vi "Do Core.vi"(8 "error in":errorcluster, 9 "Actor in":refnum<class "Actor.lvclass">, 11 "Reply Message":refnum<class "Get N Images Msg.lvclass">) -> (0 "error out":errorcluster, 1 "Actor out":refnum<class "Actor.lvclass">, 2 "Reply":refnum<class "Generic Image.lvclass">[](array[class]))   [LabVIEW 2024, in "Camera Worker.lvlib" / "Get N Images Msg.lvclass"]
doc: "<p>(<strong>Filename</strong>: <span class=\"dnl\">Actor Framework.lvlib:Reply Msg.lvclass:Do Core.vi</span>)</p>\n<p>Defines what an actor does when it receives <strong>Reply Message</strong>. This method also defines the <strong>Reply</strong> that is returned to the actor that sent <strong>Reply Message</strong>.</p>\n<p>By default, this method does nothing, and <strong>Reply</strong> is the ancestor Message class. A child class must override this method to define behavior and specify a child of the Message class to return in the <strong>Reply</strong> output.</p>"
uses:
  Get N Images Msg.lvclass
  <vilib>/ActorFramework/Actor/Actor.lvclass
  Typedefs/Generic Image/Generic Image.lvclass
  Camera Worker/Camera Worker.lvclass
  Get N Images Msg.lvclass/Get N Images Msg.ctl
  d6385fab-ef94-4aba-809e-6d8efcf0c2cc.vi
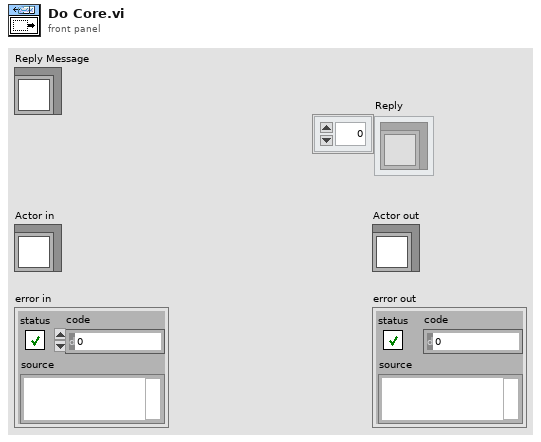
[diagram p1: front panel]
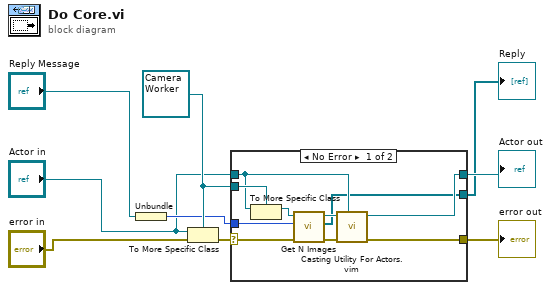
[diagram p0: block diagram]
diagram:
  w8 = refnum<class "Camera Worker.lvclass"> refnum ("Actor in")
  n1 = Unbundle("Reply Message") -> (w7:i32)
  n2 = To More Specific Class(target class=w8, reference="Actor in", error in="error in") -> (error out=w9:errorcluster)  [unwired: 1 out]
  n3 = case shown="No Error" w9 {
    selector: w9 -> [w19 w21]
    tunnel: [w13 w21] -> w2
    tunnel: [w14 w20] -> w3
    tunnel: "Actor in" -> [w16 w20]
    tunnel: w8 -> [w17 _]
    tunnel: w7 -> [w11 _]
    tunnel: [w10 _] -> w1
    frame No Error {
      n4 = To More Specific Class(target class=w17, reference=w16) -> (specific class reference=w18:refnum<class "Camera Worker.lvclass">)  [unwired: 1 in, 1 out]
      n5 = call-dynamic "Get N Images.vi"("error in"=w19, "count (-1 = all)"=w11, "Worker in"=w18) -> ("error out"=w12:errorcluster, "IImages"=w10:refnum<class "Generic Image.lvclass">[], "Worker out"=w15:refnum<class "Camera Worker.lvclass">)  [unwired: 6 in]
      n6 = call "Casting Utility For Actors.vim"("type"=w16, "error in (no error)"=w12, "Actor in"=w15) -> ("error out"=w13:errorcluster, "Actor out"=w14:refnum<class "Actor.lvclass">)  [unwired: 7 in]
    }
    frame Error {
      # "If type check fails, pass the original object out again."
    }
  }
  "error out" <- w2
  "Actor out" <- w3
  "Reply" <- w1
